vi "File - Load Controls from INI.vi"(7 "Section":string, 8 "error in (no error)":errorcluster, 9 "Array of References":refnum<vi>[](array[refnum]), 11 "INI File":path) -> (0 "error out":errorcluster)   [LabVIEW 2020]
doc: "Updates the values of controls (passed as an array of references) with the values read from an INI file.\n\nThe control names are used for the key names (with spaces removed).\n\nWorks with digital/boolean/string/path/VISAResourceName and single level clusters."
uses:
  <vilib>/Utility/config.llb/Read Key (Double).vi
  <vilib>/Utility/config.llb/Read Key (String).vi
  <vilib>/Utility/config.llb/NI_LVConfig.lvlib
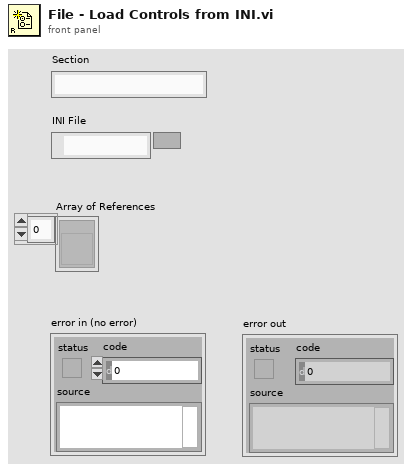
[diagram p1: front panel]
types:
  T1 = typedef "NI_LVConfig.lvlib/Config Data RefNum.ctl" = refnum<k1>
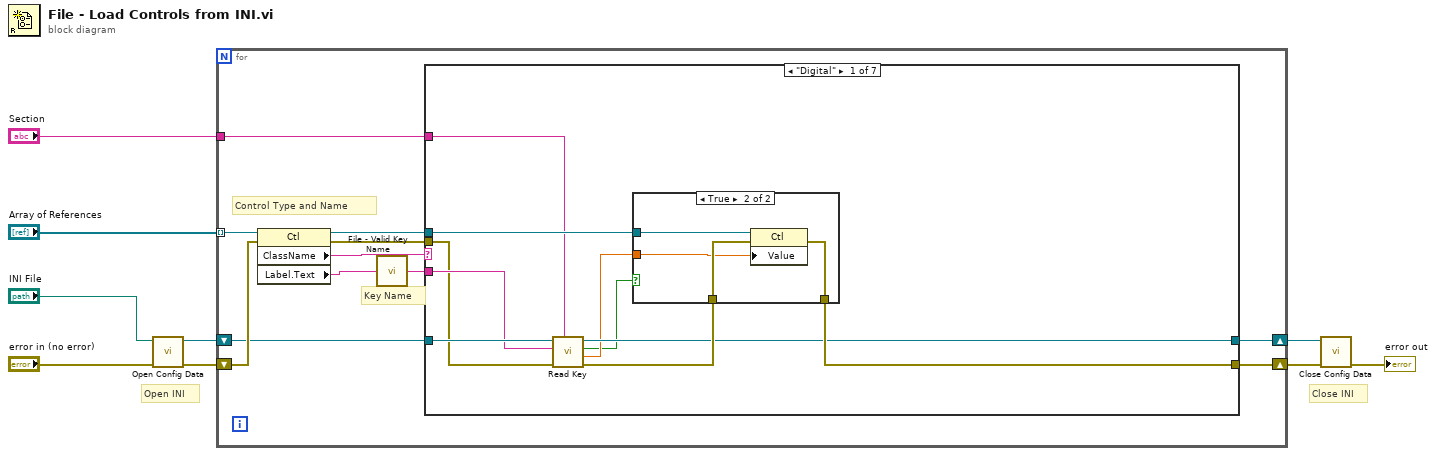
[diagram p0: block diagram]
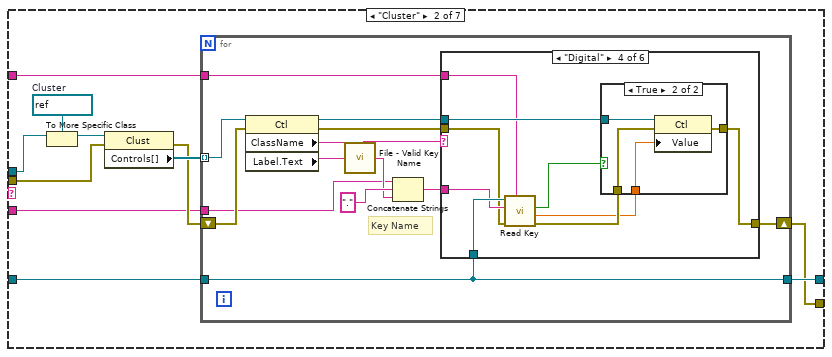
[diagram p3: hidden frame]
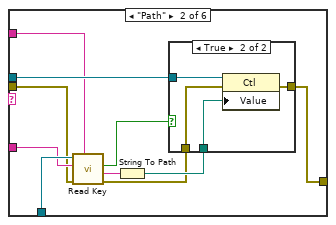
[diagram p5: hidden frame]
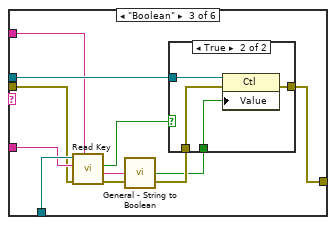
[diagram p7: hidden frame]
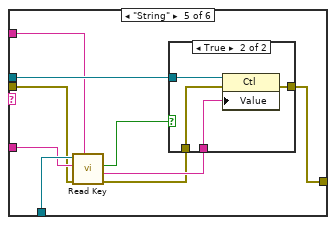
[diagram p10: hidden frame]
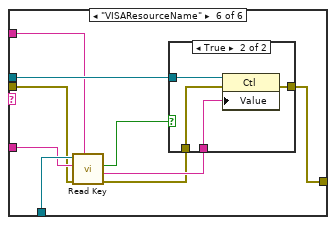
[diagram p12: hidden frame]
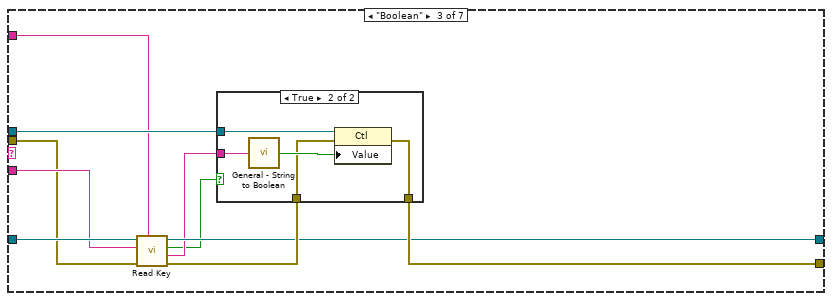
[diagram p14: hidden frame]
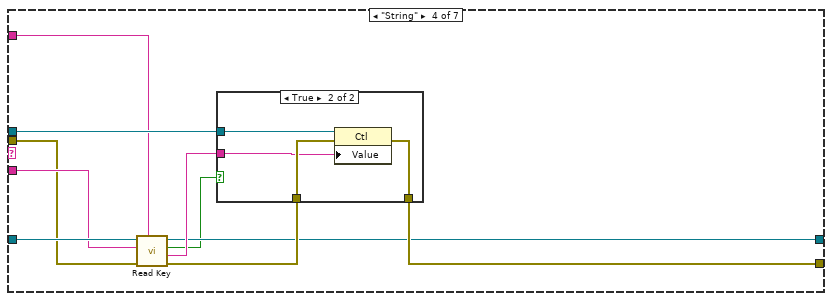
[diagram p16: hidden frame]
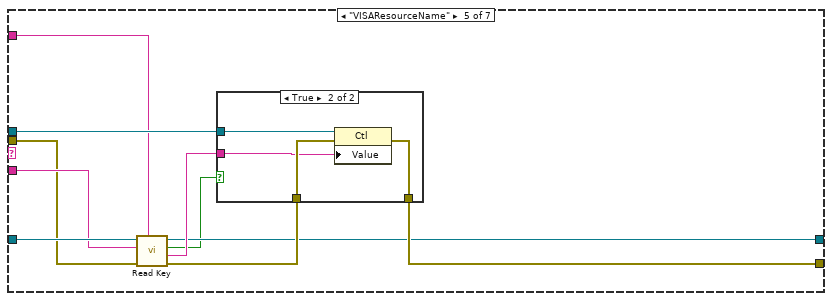
[diagram p18: hidden frame]
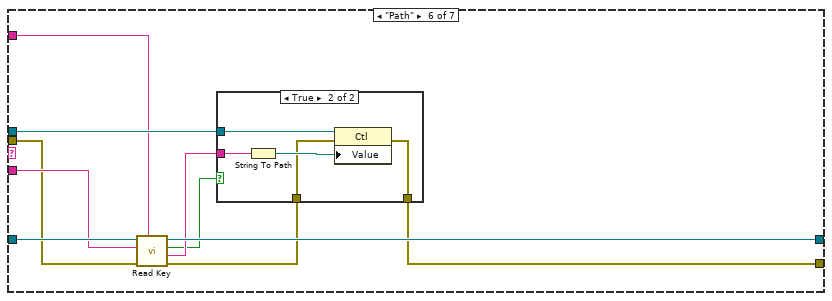
[diagram p20: hidden frame]
diagram:
  # "Close INI"
  # "Open INI"
  n1 = call <vilib>:"Open Config Data.vi"("error in (no error)"="error in (no error)", "configuration file path"="INI File") -> ("error out"=w6:errorcluster, "refnum"=w5:T1)  [unwired: 7 in, 1 out]
  n2 = for {
    tunnel: "Array of References" -> [w20] mode=indexing
    tunnel: "Section" -> [w17]
    shift-right: [w16] -> w3
    shift-left: w6 -> [w15]
    shift-right: [w13] -> w1
    shift-left: w5 -> [w14]
    # "Key Name"
    # "Control Type and Name"
    n3 = property class="Ctl"(reference=w20, error in=w15) -> (reference out=w18:refnum<vi>, error out=w10:errorcluster, "ClassName"=w19:string, "Label.Text"=w11:string)
    n4 = call "File - Valid Key Name.vi"("Key Name In"=w11) -> ("Key Name Out"=w12:string)  [unwired: 4 in]
    n5 = case shown="\"Digital\"" w19 {
      tunnel: w18 -> [w30 w44 w142 w158 w173 w188 _]
      tunnel: w12 -> [w22 w38 w134 w150 w165 w180 _]
      tunnel: w17 -> [w25 w37 w140 w155 w170 w184 _]
      tunnel: [w29 w36 w141 w157 w172 w182 w195] -> w16
      tunnel: w14 -> [w27 w43 w138 w153 w168 w186 w196]
      tunnel: [w26 w42 w137 w152 w167 w187 w196] -> w13
      tunnel: w10 -> [w21 w41 w133 w149 w164 w179 w195]
      frame "Digital" {
        n6 = call-poly <vilib>:"Read Key.vi"("section"=w25, "error in (no error)"=w21, "key"=w22, "refnum"=w27) -> ("error out"=w28:errorcluster, "value"=w24:dbl, "found?"=w23:bool, "refnum out"=w26:T1)  [unwired: 4 in]
        n7 = case shown="True" w23 {
          tunnel: w30 -> [_ w35]
          tunnel: [w31 w34] -> w29
          tunnel: w28 -> [w31 w33]
          tunnel: w24 -> [_ w32]
          frame False {
          }
          frame True {
            n8 = property class="Ctl"(reference=w35, error in=w33, "Value"=w32) -> (error out=w34:errorcluster)  [unwired: 1 out]
          }
        }
      }
      frame "Cluster" {
        w46 = refnum<vi> refnum  # Cluster
        n9 = To More Specific Class(target class=w46, reference=w44) -> (specific class reference=w45:refnum<vi>)  [unwired: 1 in, 1 out]
        n10 = property class="Clust"(reference=w45, error in=w41) -> (error out=w39:errorcluster, "Controls[]"=w40:refnum<vi>[])  [unwired: 1 out]
        n11 = for {
          tunnel: w43 -> [w50]
          tunnel: [w50] -> w42
          tunnel: w40 -> [w59] mode=indexing
          shift-right: [w47] -> w36
          shift-left: w39 -> [w58]
          tunnel: w38 -> [w54]
          tunnel: w37 -> [w49]
          # "Key Name"
          n12 = property class="Ctl"(reference=w59, error in=w58) -> (reference out=w53:refnum<vi>, error out=w48:errorcluster, "ClassName"=w51:string, "Label.Text"=w55:string)
          n13 = call "File - Valid Key Name.vi"("Key Name In"=w55) -> ("Key Name Out"=w56:string)  [unwired: 4 in]
          n14 = Concatenate Strings(w54, ".", w56) -> (w52:string)
          n15 = case shown="\"Digital\"" w51 {
            tunnel: w53 -> [_ w70 w85 w99 w113 w127]
            tunnel: w52 -> [_ w65 w82 w96 w110 w124]
            tunnel: w50 -> [_ w69 w84 w98 w112 w126]
            tunnel: w49 -> [_ w64 w81 w95 w109 w123]
            tunnel: w48 -> [w60 w63 w80 w94 w108 w122]
            tunnel: [w60 w61 w78 w92 w105 w119] -> w47
            frame Default {
            }
            frame "Path" {
              n16 = call-poly <vilib>:"Read Key.vi"("section"=w64, "error in (no error)"=w63, "key"=w65, "refnum"=w69) -> ("error out"=w62:errorcluster, "value"=w67:string, "found?"=w66:bool)  [unwired: 4 in, 1 out]
              n17 = String To Path(string=w67) -> (path=w68:path)
              n18 = case shown="True" w66 {
                tunnel: w70 -> [_ w75]
                tunnel: w68 -> [_ w74]
                tunnel: [w71 w73] -> w61
                tunnel: w62 -> [w71 w72]
                frame False {
                }
                frame True {
                  n19 = property class="Ctl"(reference=w75, error in=w72, "Value"=w74) -> (error out=w73:errorcluster)  [unwired: 1 out]
                }
              }
            }
            frame "Boolean" {
              n20 = call-poly <vilib>:"Read Key.vi"("section"=w81, "error in (no error)"=w80, "key"=w82, "refnum"=w84) -> ("error out"=w79:errorcluster, "value"=w77:string, "found?"=w83:bool)  [unwired: 4 in, 1 out]
              n21 = call "General - String to Boolean.vi"("Text In"=w77) -> ("Boolean Out"=w76:bool)  [unwired: 4 in]
              n22 = case shown="True" w83 {
                tunnel: w85 -> [_ w90]
                tunnel: w76 -> [_ w89]
                tunnel: [w86 w88] -> w78
                tunnel: w79 -> [w86 w87]
                frame False {
                }
                frame True {
                  n23 = property class="Ctl"(reference=w90, error in=w87, "Value"=w89) -> (error out=w88:errorcluster)  [unwired: 1 out]
                }
              }
            }
            frame "Digital" {
              n24 = call-poly <vilib>:"Read Key.vi"("section"=w95, "error in (no error)"=w94, "key"=w96, "refnum"=w98) -> ("error out"=w93:errorcluster, "value"=w91:dbl, "found?"=w97:bool)  [unwired: 4 in, 1 out]
              n25 = case shown="True" w97 {
                tunnel: w99 -> [_ w104]
                tunnel: w91 -> [_ w103]
                tunnel: [w100 w102] -> w92
                tunnel: w93 -> [w100 w101]
                frame False {
                }
                frame True {
                  n26 = property class="Ctl"(reference=w104, error in=w101, "Value"=w103) -> (error out=w102:errorcluster)  [unwired: 1 out]
                }
              }
            }
            frame "String" {
              n27 = call-poly <vilib>:"Read Key.vi"("section"=w109, "error in (no error)"=w108, "key"=w110, "refnum"=w112) -> ("error out"=w106:errorcluster, "value"=w107:string, "found?"=w111:bool)  [unwired: 4 in, 1 out]
              n28 = case shown="True" w111 {
                tunnel: w113 -> [_ w118]
                tunnel: w107 -> [_ w117]
                tunnel: w106 -> [w114 w116]
                tunnel: [w114 w115] -> w105
                frame False {
                }
                frame True {
                  n29 = property class="Ctl"(reference=w118, error in=w116, "Value"=w117) -> (error out=w115:errorcluster)  [unwired: 1 out]
                }
              }
            }
            frame "VISAResourceName" {
              n30 = call-poly <vilib>:"Read Key.vi"("section"=w123, "error in (no error)"=w122, "key"=w124, "refnum"=w126) -> ("error out"=w120:errorcluster, "value"=w121:string, "found?"=w125:bool)  [unwired: 4 in, 1 out]
              n31 = case shown="True" w125 {
                tunnel: w127 -> [_ w132]
                tunnel: w121 -> [_ w131]
                tunnel: w120 -> [w128 w130]
                tunnel: [w128 w129] -> w119
                frame False {
                }
                frame True {
                  n32 = property class="Ctl"(reference=w132, error in=w130, "Value"=w131) -> (error out=w129:errorcluster)  [unwired: 1 out]
                }
              }
            }
          }
        }
      }
      frame "Boolean" {
        n33 = call-poly <vilib>:"Read Key.vi"("section"=w140, "error in (no error)"=w133, "key"=w134, "refnum"=w138) -> ("error out"=w139:errorcluster, "value"=w136:string, "found?"=w135:bool, "refnum out"=w137:T1)  [unwired: 4 in]
        n34 = case shown="True" w135 {
          tunnel: w142 -> [_ w148]
          tunnel: [w143 w146] -> w141
          tunnel: w139 -> [w143 w145]
          tunnel: w136 -> [_ w144]
          frame False {
          }
          frame True {
            n35 = call "General - String to Boolean.vi"("Text In"=w144) -> ("Boolean Out"=w147:bool)  [unwired: 4 in]
            n36 = property class="Ctl"(reference=w148, error in=w145, "Value"=w147) -> (error out=w146:errorcluster)  [unwired: 1 out]
          }
        }
      }
      frame "String" {
        n37 = call-poly <vilib>:"Read Key.vi"("section"=w155, "error in (no error)"=w149, "key"=w150, "refnum"=w153) -> ("error out"=w156:errorcluster, "value"=w154:string, "found?"=w151:bool, "refnum out"=w152:T1)  [unwired: 4 in]
        n38 = case shown="True" w151 {
          tunnel: w158 -> [_ w163]
          tunnel: [w159 w162] -> w157
          tunnel: w156 -> [w159 w161]
          tunnel: w154 -> [_ w160]
          frame False {
          }
          frame True {
            n39 = property class="Ctl"(reference=w163, error in=w161, "Value"=w160) -> (error out=w162:errorcluster)  [unwired: 1 out]
          }
        }
      }
      frame "VISAResourceName" {
        n40 = call-poly <vilib>:"Read Key.vi"("section"=w170, "error in (no error)"=w164, "key"=w165, "refnum"=w168) -> ("error out"=w171:errorcluster, "value"=w169:string, "found?"=w166:bool, "refnum out"=w167:T1)  [unwired: 4 in]
        n41 = case shown="True" w166 {
          tunnel: w173 -> [_ w178]
          tunnel: [w174 w177] -> w172
          tunnel: w171 -> [w174 w176]
          tunnel: w169 -> [_ w175]
          frame False {
          }
          frame True {
            n42 = property class="Ctl"(reference=w178, error in=w176, "Value"=w175) -> (error out=w177:errorcluster)  [unwired: 1 out]
          }
        }
      }
      frame "Path" {
        n43 = call-poly <vilib>:"Read Key.vi"("section"=w184, "error in (no error)"=w179, "key"=w180, "refnum"=w186) -> ("error out"=w183:errorcluster, "value"=w185:string, "found?"=w181:bool, "refnum out"=w187:T1)  [unwired: 4 in]
        n44 = case shown="True" w181 {
          tunnel: w188 -> [_ w194]
          tunnel: w185 -> [_ w192]
          tunnel: w183 -> [w189 w191]
          tunnel: [w189 w190] -> w182
          frame False {
          }
          frame True {
            n45 = String To Path(string=w192) -> (path=w193:path)
            n46 = property class="Ctl"(reference=w194, error in=w191, "Value"=w193) -> (error out=w190:errorcluster)  [unwired: 1 out]
          }
        }
      }
      frame Default {
      }
    }
  }
  n47 = call <vilib>:"Close Config Data.vi"("error in (no error)"=w3, "refnum"=w1) -> ("error out"=→"error out":errorcluster)  [unwired: 8 in, 1 out]
